vi "Unreserve.vi"(8 "error in (no error)":errorcluster, 9 "Sequence Parameters in":variant, 11 "Step in":refnum<class "Step.lvclass">) -> (0 "error out":errorcluster, 1 "Sequence Parameters out":variant, 3 "Step out":refnum<class "Step.lvclass">)   [LabVIEW 2015, in "Mediator.lvlib" / "Step.lvclass"]
doc: "This unreserves any resources used by this step."
uses:
  Step.lvclass
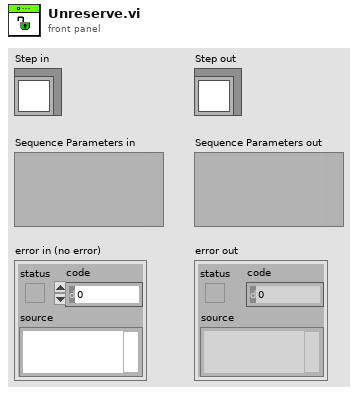
[diagram p1: front panel]
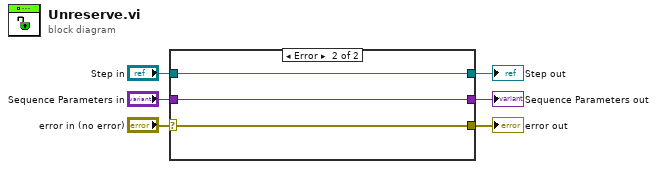
[diagram p0: block diagram]
diagram:
  n1 = case shown="Error" "error in (no error)" {
    selector: "error in (no error)" -> [w8 w12]
    tunnel: [w8 w12] -> w5
    tunnel: [w9 w11] -> w3
    tunnel: "Step in" -> [w9 w11]
    tunnel: [w7 w10] -> w2
    tunnel: "Sequence Parameters in" -> [w7 w10]
    frame No Error {
      # "Wire the error cluster across even in the \"No Error\"\ncase so that warnings get propagated."
    }
    frame Error {
    }
  }
  "error out" <- w5
  "Step out" <- w3
  "Sequence Parameters out" <- w2
